vi "Report Save.vi"(4 "Model No.":string, 5 "Data In":T1) -> ()   [LabVIEW 2015]
uses:
  <vilib>/Utility/file.llb/Write Delimited Spreadsheet (string).vi
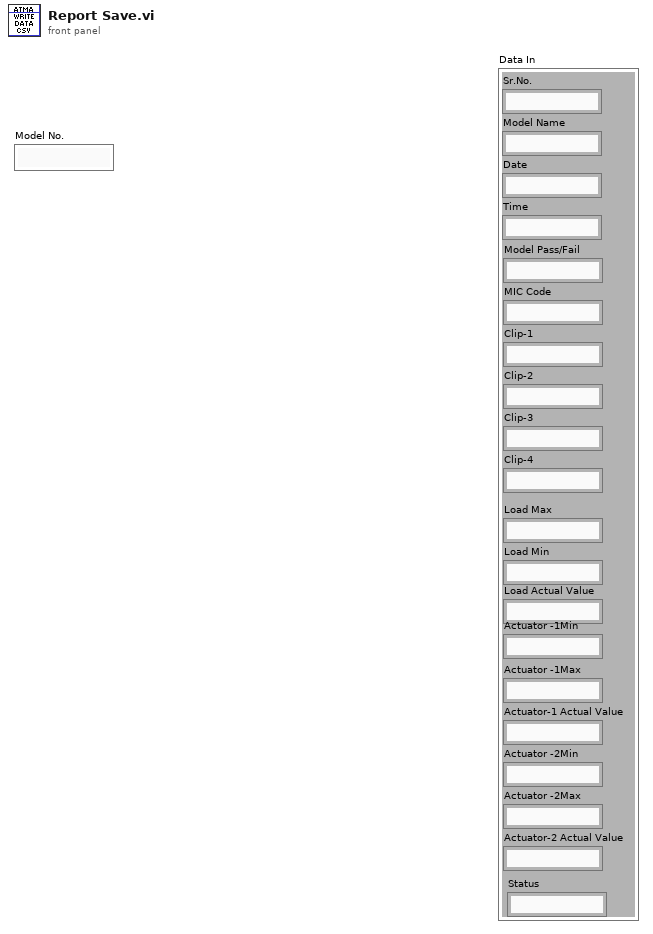
[diagram p1: front panel]
types:
  T1 = cluster{"Sr.No.":string, "Model Name":string, "Date":string, "Time":string, "Model Pass/Fail":string, "MIC Code":string, "Clip-1":string, "Clip-2":string, "Clip-3":string, "Clip-4":string, "Load Max":string, "Load Min":string, "Load Actual Value":string, "Actuator -1Min":string, "Actuator -1Max":string, "Actuator-1 Actual Value":string, "Actuator -2Min ":string, "Actuator -2Max ":string, "Actuator-2 Actual Value ":string, "Status":string}
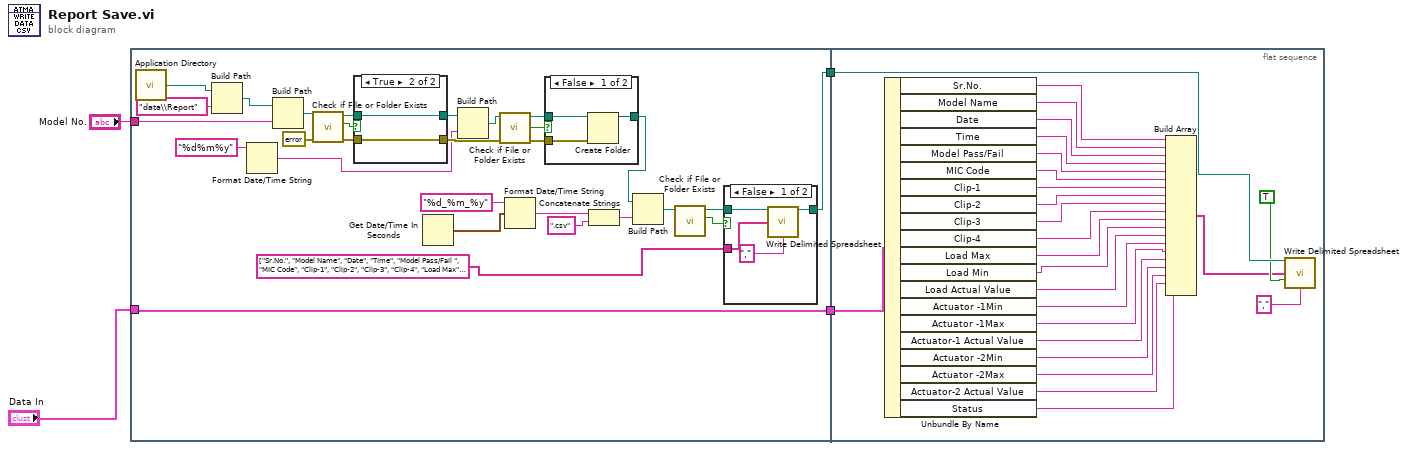
[diagram p0: block diagram]
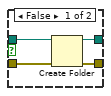
[diagram p3: hidden frame]
diagram:
  n1 = flat-sequence {
    tunnel: [w25] -> w4
    tunnel: [w16] -> w3
    tunnel: "Data In" -> [w16]
    tunnel: "Model No." -> [w15]
    tunnel: w4 -> [w60]
    tunnel: w3 -> [w64]
    frame #0 {
      n2 = call <vilib>:"Application Directory.vi"() -> ("Application Directory"=w23:path)
      n3 = Build Path(base path=w23, name or relative path="data\\Report") -> (appended path=w18:path)
      n4 = Format Date/Time String(time format string (%c)="%d%m%y") -> (date/time string=w8:string)  [unwired: 2 in]
      n5 = Build Path(base path=w18, name or relative path=w15) -> (appended path=w17:path)
      n6 = call <vilib>:"Check if File or Folder Exists.vi"("error in (no error)"=errorcluster {"status"=FALSE, "code"=0, "source"=""}, "path"=w17) -> ("error out"=w21:errorcluster, "file or folder exists?"=w19:bool, "dup path"=w22:path)  [unwired: 7 in]
      n7 = case shown="True" w19 {
        tunnel: w22 -> [w41 w43]
        tunnel: [w40 w43] -> w9
        tunnel: w21 -> [w39 w42]
        tunnel: [w38 w42] -> w10
        frame False {
          n8 = Create Folder(path (use dialog)=w41, error in=w39) -> (created path=w40:path, error out=w38:errorcluster)  [unwired: 1 in, 1 out]
        }
        frame True {
        }
      }
      n9 = Get Date/Time In Seconds() -> (seconds since 1Jan1904=w31:timestamp)
      n10 = Build Path(base path=w9, name or relative path=w8) -> (appended path=w7:path)
      n11 = call <vilib>:"Check if File or Folder Exists.vi"("error in (no error)"=w10, "path"=w7) -> ("error out"=w12:errorcluster, "file or folder exists?"=w13:bool, "dup path"=w11:path)  [unwired: 7 in]
      n12 = Format Date/Time String(time format string (%c)="%d_%m_%y", seconds (now)=w31) -> (date/time string=w29:string)  [unwired: 1 in]
      n13 = case shown="False" w13 {
        tunnel: w11 -> [w36 w37]
        tunnel: [w35 w37] -> w6
        tunnel: w12 -> [w34 _]
        frame False {
          n14 = Create Folder(path (use dialog)=w36, error in=w34) -> (created path=w35:path)  [unwired: 1 in, 2 out]
        }
        frame True {
        }
      }
      n15 = Concatenate Strings(w29, ".csv" ("string")) -> (w27:string)
      n16 = Build Path(base path=w6, name or relative path=w27) -> (appended path=w26:path)
      n17 = call <vilib>:"Check if File or Folder Exists.vi"("path"=w26) -> ("file or folder exists?"=w33:bool, "dup path"=w32:path)  [unwired: 8 in, 1 out]
      n18 = case shown="False" w33 {
        tunnel: [w44 w48] -> w25
        tunnel: w32 -> [w46 w48]
        tunnel: string[] ["Sr.No.", "Model Name", "Date", "Time", "Model Pass/Fail ", "MIC Code", "Clip-1", "Clip-2", "Clip-3", "Clip-4", "Load Max", "Load Min", "Load Actual Value", "Actuator-1 Min", "Actuator-1 Max", "Actuator-1 Actual Value", "Actuator-2 Min", "Actuator-2 Max", "Actuator-2 Actual Value", "Status"] ("Array") -> [w45 _]
        frame False {
          n19 = call-poly <vilib>:"Write Delimited Spreadsheet.vi"("file path (dialog if empty)"=w46, "1D data"=w45, "delimiter (\\t)"="," ("delimiter (\\t)")) -> ("new file path (Not A Path if cancelled)"=w44:path)  [unwired: 11 in, 1 out]
        }
        frame True {
        }
      }
    }
    frame #1 {
      n20 = Unbundle By Name(w64) -> ("Sr.No."=w65:string, "Model Name"=w66:string, "Date"=w67:string, "Time"=w68:string, "Model Pass/Fail"=w69:string, "MIC Code"=w70:string, "Clip-1"=w71:string, "Clip-2"=w72:string, "Clip-3"=w73:string, "Clip-4"=w63:string, "Load Max"=w62:string, "Load Min"=w57:string, "Load Actual Value"=w56:string, "Actuator -1Min"=w55:string, "Actuator -1Max"=w54:string, "Actuator-1 Actual Value"=w53:string, "Actuator -2Min"=w52:string, "Actuator -2Max"=w51:string, "Actuator-2 Actual Value"=w50:string, "Status"=w49:string)
      n21 = Build Array(w65, w66, w67, w68, w69, w70, w71, w72, w73, w63, w62, w57, w56, w55, w54, w53, w52, w51, w50, w49) -> (w58:string[])
      n22 = call-poly <vilib>:"Write Delimited Spreadsheet.vi"("file path (dialog if empty)"=w60, "1D data"=w58, "append to file? (F)"=TRUE, "delimiter (\\t)"="," ("delimiter (\\t)")) -> ()  [unwired: 10 in, 2 out]
    }
  }
